vi "(Sub VI) Parse move T.vi"(11 "data":string) -> (2 "Motion parameters":T1, 3 "Position T":T5 {"Az" format="%.4f"; "Ay" format="%.4f"; "Ax" format="%.4f"; "Oz" format="%.4f"; "Oy" format="%.4f"; "Ox" format="%.4f"; "Z" format="%.4f"; "Y" format="%.4f"; "X" format="%.4f"})   [LabVIEW 2022 SP3]
uses:
  <vilib>/ImagingLab/Denso Robotics Library/_Private/Controls/drl_Variable T.ctl
  <vilib>/ImagingLab/Denso Robotics Library/DensoRoboticsLibrary.lvlib
  <vilib>/ImagingLab/Denso Robotics Library/_Private/Controls/drl_Interpolation.ctl
  <vilib>/ImagingLab/Denso Robotics Library/_Private/Controls/drl_Pass motion.ctl
  <vilib>/ImagingLab/Denso Robotics Library/_Private/Controls/drl_Move option.ctl
  <vilib>/ImagingLab/Denso Robotics Library/_Private/Controls/drl_Motion parameters.ctl
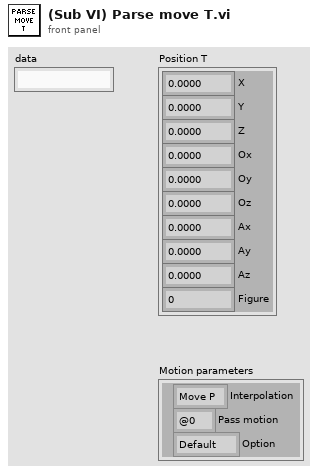
[diagram p1: front panel]
types:
  T1 = typedef "DensoRoboticsLibrary.lvlib/drl_Motion parameters.ctl" = cluster{"Interpolation":T2, "Pass motion":T3, "Option":T4}
  T2 = typedef "DensoRoboticsLibrary.lvlib/drl_Interpolation.ctl" = enum16{"Move P", "Move L"}
  T3 = typedef "DensoRoboticsLibrary.lvlib/drl_Pass motion.ctl" = enum16{"@0", "@P", "@E"}
  T4 = typedef "DensoRoboticsLibrary.lvlib/drl_Move option.ctl" = enum16{"Default", "Next"}
  T5 = typedef "DensoRoboticsLibrary.lvlib/drl_Variable T.ctl" = cluster{"X":sgl, "Y":sgl, "Z":sgl, "Ox":sgl, "Oy":sgl, "Oz":sgl, "Ax":sgl, "Ay":sgl, "Az":sgl, "Figure":sgl}
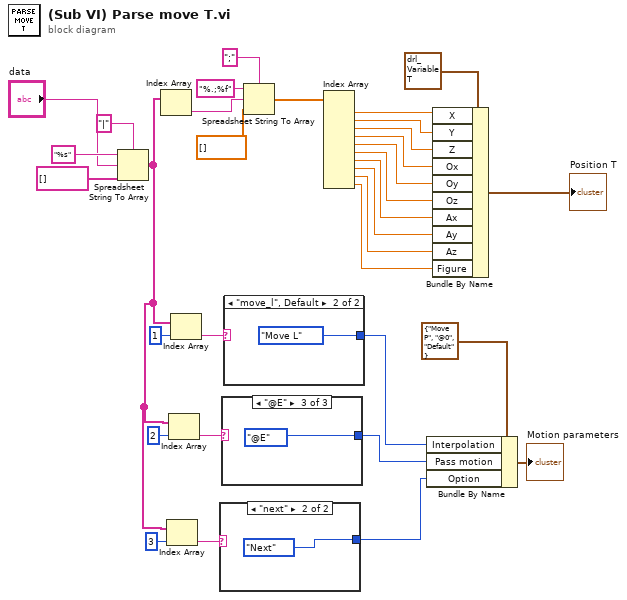
[diagram p0: block diagram]
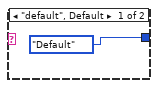
[diagram p2: hidden frame]
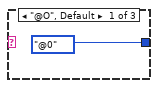
[diagram p3: hidden frame]
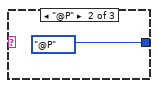
[diagram p4: hidden frame]
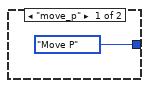
[diagram p5: hidden frame]
diagram:
  n1 = Spreadsheet String To Array(delimiter (Tab)="|", format string="%s", spreadsheet string="data", array type (2D Dbl)=string[] []) -> (array=w28:string[])
  n2 = Index Array(array=w28) -> (element=w21:string)  [unwired: 1 in]
  n3 = Index Array(array=w28, index=3) -> (element=w26:string)
  n4 = Index Array(array=w28, index=2) -> (element=w25:string)
  n5 = Index Array(array=w28, index=1) -> (element=w22:string)
  n6 = case shown="\"next\"" w26 {
    tunnel: [drl_Move_option."Default" ("Option") drl_Move_option."Next" ("Option")] -> w31
    frame "default", Default {
    }
    frame "next" {
    }
  }
  n7 = case shown="\"@E\"" w25 {
    tunnel: [drl_Pass_motion."@0" ("Pass motion") drl_Pass_motion."@P" ("Pass motion") drl_Pass_motion."@E" ("Pass motion")] -> w30
    frame "@O", Default {
    }
    frame "@P" {
    }
    frame "@E" {
    }
  }
  n8 = case shown="\"move_l\", Default" w22 {
    tunnel: [drl_Interpolation."Move P" ("Interpolation") drl_Interpolation."Move L" ("Interpolation")] -> w29
    frame "move_p" {
    }
    frame "move_l", Default {
    }
  }
  n9 = Spreadsheet String To Array(delimiter (Tab)=";", format string="%.;%f", spreadsheet string=w21, array type (2D Dbl)=dbl[] []) -> (array=w4:dbl[])
  n10 = Index Array(array=w4) -> (element #1=w6:dbl, element #2=w7:dbl, element #3=w8:dbl, element #4=w9:dbl, element #5=w10:dbl, element #6=w11:dbl, element #7=w12:dbl, element #8=w13:dbl, element #9=w14:dbl, element #10=w15:dbl)  [unwired: 10 in]
  n11 = Bundle By Name(cluster=T1 {"Interpolation"=enum."Move P", "Pass motion"=enum."@0", "Option"=enum."Default"} ("motion parameters"), "Interpolation"=w29, "Pass motion"=w30, "Option"=w31) -> (→"Motion parameters":T1)
  n12 = Bundle By Name(cluster=T5 {"X"=0.0, "Y"=0.0, "Z"=0.0, "Ox"=0.0, "Oy"=0.0, "Oz"=0.0, "Ax"=0.0, "Ay"=0.0, "Az"=0.0, "Figure"=0.0} ("position T"), "X"=w6, "Y"=w7, "Z"=w8, "Ox"=w9, "Oy"=w10, "Oz"=w11, "Ax"=w12, "Ay"=w13, "Az"=w14, "Figure"=w15) -> (→"Position T":T5)
